vi "Daq Port & Line.vi"(1 "Daq Setting":string[](array[string])) -> (0 "DAQ Port &line":tag)   [LabVIEW 2015]
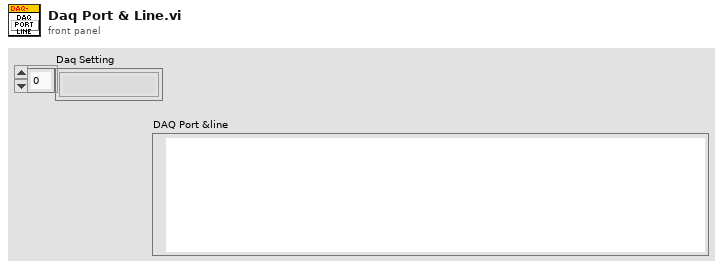
[diagram p1: front panel]
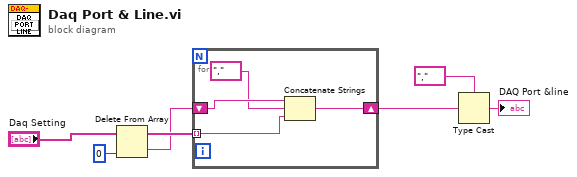
[diagram p0: block diagram]
diagram:
  n1 = Delete From Array(array="Daq Setting", index=0) -> (deleted portion=w5:string, array with subset deleted=w7:string[])  [unwired: 1 in]
  n2 = for {
    tunnel: w7 -> [w10] mode=indexing
    shift-right: [w8] -> w3
    shift-left: w5 -> [w11]
    n3 = Concatenate Strings(w11, tag "," ("1."), w10) -> (w8:string)
  }
  n4 = Type Cast(type=tag "," ("1."), x=w3) -> (*(type *) &x=→"DAQ Port &line":tag)
